vi "Background.vi"(5 "Image data max":dbl(slide)=63.63636363636363 min=0.0 max=100.0 scale=0.0..100.0, 7 "Image data min":dbl(slide)=61.832061068702295 min=0.0 max=100.0 scale=0.0..100.0, 8 "error in (no error)":errorcluster, 9 "Resolution":i32=444, 10 "Page":i32=1, 11 "Image File Path":path=path "P:/users1/Yun-Yi Pai/Devices/SA02775/20160403/SA02775G0001.ibw") -> (0 "error out":errorcluster, 1 "Max Pages":i32, 2 "Corrected Page":i32=1, 3 "Background out":T1)   [LabVIEW 2019]
doc: "This VI loads the background image from a file into an IMAQ image and sets the resolution."
uses:
  <vilib>/vision/Image Controls.llb/IMAQ Image.ctl
  <vilib>/vision/NI_Vision_Development_Module.lvlib
  <vilib>/Utility/sysdir.llb/System Directory Type.ctl
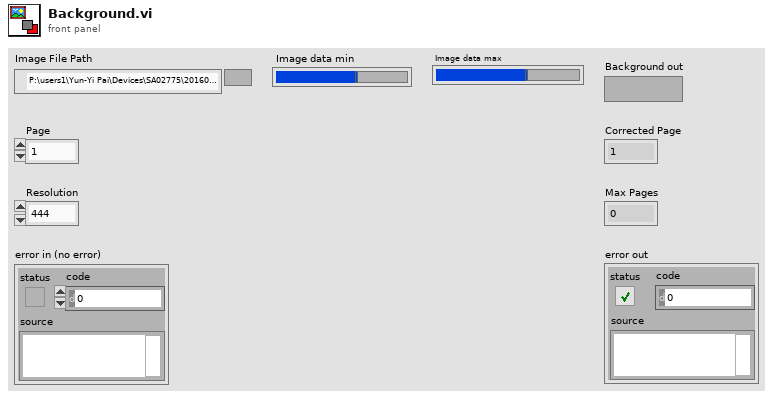
[diagram p1: front panel]
types:
  T1 = typedef "IMAQ Image.ctl" = refnum<image>
  T2 = typedef "Image Type" = u32
  T3 = typedef "System Directory Type.ctl" = i32
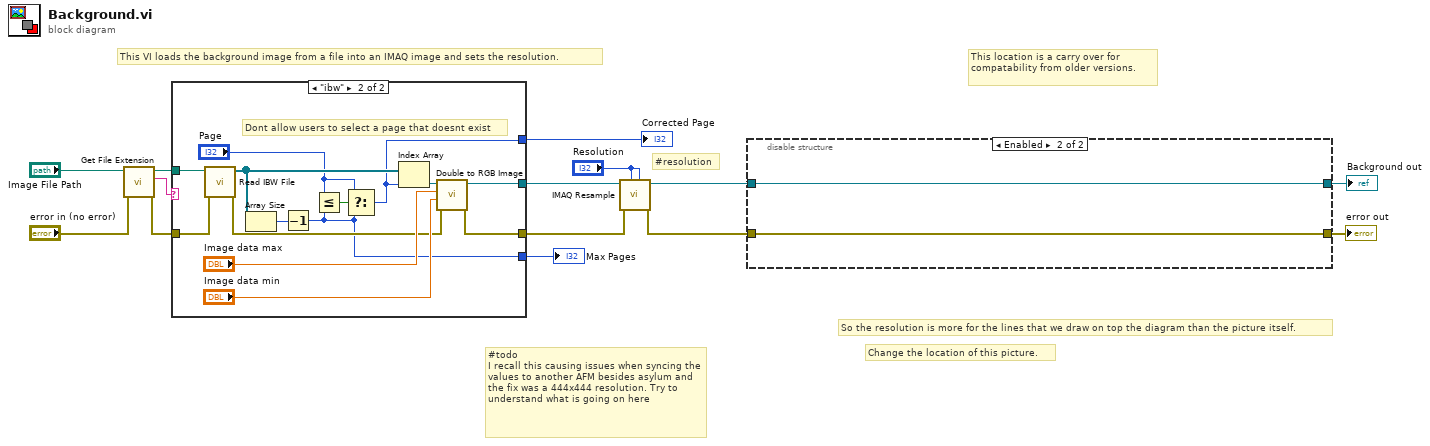
[diagram p0: block diagram]
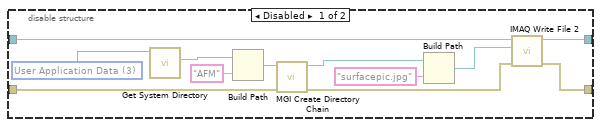
[diagram p2: hidden frame]
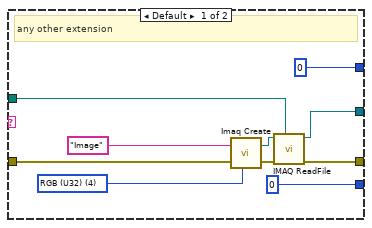
[diagram p3: hidden frame]
diagram:
  # "This location is a carry over for compatability from older versions."
  # "Change the location of this picture."
  # "So the resolution is more for the lines that we draw on top the diagram than the picture itself."
  # "#resolution"
  # "#todo \nI recall this causing issues when syncing the values to another AFM besides asylum and the fix was a 444x444 resolution. Try to understand what is going on here"
  # "This VI loads the background image from a file into an IMAQ image and sets the resolution."
  n1 = call <vilib>:"Get File Extension.vi"("error in (no error)"="error in (no error)", "file"="Image File Path") -> ("error out"=w11:errorcluster, "lowercase file extension"=w14:string, "dup file"=w12:path)  [unwired: 5 in, 2 out]
  n2 = case shown="\"ibw\"" w14 {
    tunnel: [w24 w38] -> w5
    tunnel: [w23 w28] -> w2
    tunnel: w12 -> [w17 w35]
    tunnel: w11 -> [w18 w32]
    tunnel: [0 w27] -> w7
    tunnel: [0 ("Page") w25] -> w4
    frame Default {
      w22 = T2 4 items=["Grayscale (U8)", "Grayscale (I16)", "Grayscale (SGL)", "Complex (CSG)", "RGB (U32)", "HSL (U32)", "RGB (U64)", "Grayscale (U16)"] ("Image Type")
      # "any other extension"
      n3 = call "Imaq Create"("Image Name"="Image", "Image Type"=w22, "error in (no error)"=w18) -> ("New Image"=w19:T1, "error out"=w20:errorcluster)  [unwired: 2 in]
      n4 = call "IMAQ ReadFile"("File Path"=w17, "error in (no error)"=w20, "Image"=w19) -> ("error out"=w23:errorcluster, "Image Out"=w24:T1)  [unwired: 4 in, 3 out]
    }
    frame "ibw" {
      # "Dont allow users to select a page that doesnt exist"
      n5 = call "Read IBW File.vi"("error in (no error)"=w32, "Path"=w35) -> ("error out"=w33:errorcluster, "IMAQ"=w31:T1[])  [unwired: 7 in, 1 out]
      n6 = Array Size(array=w31) -> (size(s)=w30:i32)
      n7 = Decrement(x=w30) -> (x-1=w27:i32)
      n8 = Less Or Equal?(x="Page", y=w27) -> (x <= y?=w29:bool)
      n9 = Select(t="Page", s=w29, f=w27) -> (s? t:f=w25:i32)
      n10 = Index Array(array=w31, index=w25) -> (element=w34:T1)
      n11 = call "Double to RGB Image.vi"("error in (no error)"=w33, "minimum"="Image data min", "maximum"="Image data max", "Image Reference In"=w34) -> ("error out"=w28:errorcluster, "Image Reference Out"=w38:T1)  [unwired: 6 in]
    }
  }
  "Max Pages" <- w7
  "Corrected Page" <- w4
  n12 = call "IMAQ Resample"("X Resolution"="Resolution", "Y Resolution"="Resolution", "error in (no error)"=w2, "Image Src"=w5) -> ("error out"=w1:errorcluster, "Image Dst Out"=w10:T1)  [unwired: 6 in]
  n13 = disable-structure shown="Enabled" {
    disable-tunnel: w10 -> [w48 w52]
    disable-tunnel: [w47 w52] -> w9
    disable-tunnel: [w45 w51] -> w8
    disable-tunnel: w1 -> [w44 w51]
    frame Disabled {
      w43 = T3 3 items=["User Home"=0, "User Desktop"=1, "User Documents"=2, "User Application Data"=3, "User Preferences"=4, "User Temporary"=5, "Public Documents"=6, "Public Application Data"=7, "Public Preferences"=8, "Public Cache"=13, "System Core Libraries"=9, "System Installed Libraries"=10, "Application Files"=11, "Boot Volume Root"=12] ("system directory type")
      n14 = call <vilib>:"Get System Directory.vi"("system directory type"=w43) -> ("system directory"=w41:path)  [unwired: 10 in]
      n15 = Build Path(base path=w41, name or relative path="AFM") -> (appended path=w39:path)
      n16 = call <userlib>:"MGI Create Directory Chain.vi"("Error In"=w44, "Path"=w39) -> ("Error Out"=w46:errorcluster, "Duplicate Path"=w49:path)  [unwired: 8 in]
      n17 = Build Path(base path=w49, name or relative path="surfacepic.jpg" ("File Path")) -> (appended path=w50:path)
      n18 = call-poly "IMAQ Write File 2"("error in (no error)"=w46, "File Path"=w50, "Image"=w48) -> ("error out"=w45:errorcluster, "Image Out (duplicate)"=w47:T1)  [unwired: 7 in]
    }
    frame Enabled {
    }
  }
  "error out" <- w8
  "Background out" <- w9
